vi "Write time.vi"(8 "error in (no error)":errorcluster, 10 "time":dbl[unit] min=0.0 max=86400.0, 11 "RotatorTracking in":refnum<class "RotatorTracking.lvclass">) -> (0 "error out":errorcluster, 3 "RotatorTracking out":refnum<class "RotatorTracking.lvclass">)   [LabVIEW 2022 SP3, in "TCSDataDefinitions.lvlib" / "TCSMountControlStatus.lvlib" / "RotatorTracking.lvclass"]
uses:
  RotatorTracking.lvclass
  RotatorTracking.lvclass/RotatorTracking.ctl
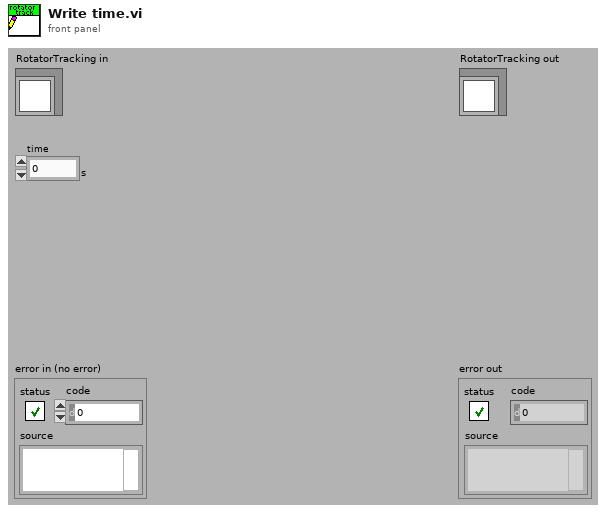
[diagram p1: front panel]
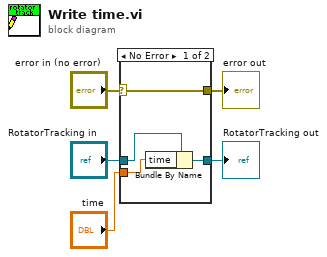
[diagram p0: block diagram]
diagram:
  n1 = case shown="No Error" "error in (no error)" {
    selector: "error in (no error)" -> [w9 w10]
    tunnel: [w9 w10] -> w4
    tunnel: [w7 w11] -> w2
    tunnel: "RotatorTracking in" -> [w8 w11]
    tunnel: "time" -> [w6 _]
    frame No Error {
      n2 = Bundle By Name(cluster=w8, "time"=w6) -> (w7:refnum<class "RotatorTracking.lvclass">)
    }
    frame Error {
    }
  }
  "error out" <- w4
  "RotatorTracking out" <- w2
